vi "MainRTLocal.vi"() -> ()   [LabVIEW 2018]
doc: "The myRIO Project template acquires acceleration data from the onboard accelerometer and displays the changes of acceleration values in a waveform chart."
uses:
  <vilib>/myRIO/Instrument Drivers/Onboard IO/DIO/typedefs/DIO Reference.ctl
  <vilib>/myRIO/Common/Instrument Driver Framework/Utilities/typedefs/myRIO Generic Hardware Reference.ctl
  <vilib>/myRIO/Common/Instrument Driver Framework/Utilities/typedefs/Hardware Version Enum.ctl
  <vilib>/myRIO/Common/Instrument Driver Framework/Utilities/typedefs/myRIO v1.0 Reference.ctl
  <vilib>/myRIO/Common/Instrument Driver Framework/Utilities/typedefs/Generic FPGA Reference.ctl
  <vilib>/myRIO/Common/Instrument Driver Framework/myRIO v1.0/DIO/typedefs/DIO Channels List.ctl
  <vilib>/myRIO/Common/Instrument Driver Framework/myRIO v1.0/DIO/typedefs/DIO Channels Enum.ctl
  <vilib>/userdefined/High Color/nirio_resource_hc.ctl
  <vilib>/myRIO/Instrument Drivers/Onboard IO/PWM/typedefs/PWM Reference.ctl
  <vilib>/myRIO/Common/Instrument Driver Framework/myRIO v1.0/PWM/typedefs/PWM Channels Enum.ctl
  <vilib>/myRIO/Instrument Drivers/Onboard IO/PWM/typedefs/PWM Configuration.ctl
  <vilib>/myRIO/Common/Instrument Driver Framework/Utilities/vis/Is FPGA Ref Available.vi
  <vilib>/myRIO/Common/Instrument Driver Framework/myRIO v1.0/DIO/vis/myRIO v1.1 Open DIO.vi
  <vilib>/myRIO/Instrument Drivers/Onboard IO/DIO/vis/Write.vi
  <vilib>/myRIO/Common/Instrument Driver Framework/myRIO v1.0/PWM/vis/myRIO v1.1 Open PWM.vi
  <vilib>/myRIO/Instrument Drivers/Onboard IO/PWM/vis/Set Duty Cycle and Frequency.vi
  <vilib>/myRIO/Common/Instrument Driver Framework/Utilities/vis/Validate Channels.vi
  <vilib>/myRIO/Common/Instrument Driver Framework/myRIO v1.0/DIO/vis/myRIO v1.0 Reserve DIO.vi
  <vilib>/myRIO/Common/Instrument Driver Framework/myRIO v1.0/PWM/vis/myRIO v1.0 Reserve PWM.vi
  <vilib>/myRIO/Common/Instrument Driver Framework/myRIO v1.0/UART/vis/myRIO v1.0 Close UART.vi
  <vilib>/myRIO/Common/Instrument Driver Framework/myRIO v1.0/Resource Manager/vis/myRIO v1.0 Reserve Channel List.vi
  <vilib>/myRIO/Common/Instrument Driver Framework/myRIO v1.0/DIO/vis/myRIO v1.0 Build MUX Configuration DIO.vi
  <vilib>/myRIO/Common/Instrument Driver Framework/myRIO v1.0/PWM/vis/myRIO v1.0 Build MUX Configuration PWM.vi
  <vilib>/myRIO/Common/Instrument Driver Framework/myRIO v1.0/Resource Manager/vis/myRIO v1.0 Reserve Channel.vi
  <vilib>/myRIO/Common/Instrument Driver Framework/myRIO v1.0/Resource Manager/vis/myRIO v1.0 Unreserve Channel.vi
  <vilib>/myRIO/Common/Instrument Driver Framework/myRIO v1.0/Resource Manager/vis/myRIO v1.0 Create Configuration List.vi
  <vilib>/myRIO/Common/Instrument Driver Framework/myRIO v1.0/Resource Manager/vis/myRIO v1.0 Build Mutex Name.vi
  <vilib>/Utility/VariantDataType/GetNumericInfo.vi
  <vilib>/Utility/error.llb/Error Cluster From Error Code.vi
  <vilib>/myRIO/Common/Instrument Driver Framework/myRIO v1.0/myRIO v1.1 Open.vi
  <vilib>/myRIO/Common/Instrument Driver Framework/Utilities/vis/IO Manager.vi
  <vilib>/myRIO/Common/Instrument Driver Framework/Utilities/vis/Configuration Manager.vi
  <vilib>/myRIO/Common/Instrument Driver Framework/myRIO v1.0/Resource Manager/vis/myRIO v1.0 Configure IO.vi
  <vilib>/myRIO/Common/Instrument Driver Framework/myRIO v1.0/myRIO v1.0 Close.vi
  <vilib>/myRIO/Common/Instrument Driver Framework/myRIO v1.0/DIO/vis/myRIO v1.0 Write DIO.vi
  <vilib>/myRIO/Common/Instrument Driver Framework/myRIO v1.0/PWM/vis/myRIO v1.0 Write PWM.vi
  <vilib>/myRIO/Common/Instrument Driver Framework/Utilities/vis/FPGA Ref Manager.vi
  <vilib>/myRIO/Common/Instrument Driver Framework/myRIO v1.0/myRIO v1.0 Reset FPGA.vi
  <vilib>/myRIO/Common/Instrument Driver Framework/myRIO v1.0/IRQ/vis/myRIO v1.0 IRQ Info FGV.vi
  <vilib>/myRIO/Common/Instrument Driver Framework/myRIO v1.0/IRQ/vis/myRIO v1.0 Timer IRQ Info FGV.vi
  <vilib>/myRIO/Common/Instrument Driver Framework/myRIO v1.0/IRQ/vis/myRIO v1.0 ISR Agent.vi
  <vilib>/myRIO/Express VI/Onboard Devices/LED/LED Express VI.xnode
  <vilib>/myRIO/Instrument Drivers/Onboard IO/DIO/vis/myRIO DIO Open.xnode
  <vilib>/myRIO/Express VI/Onboard IO/PWM/PWM Express VI.xnode
  <vilib>/myRIO/Instrument Drivers/Onboard IO/PWM/vis/myRIO PWM Open.xnode
  <vilib>/myRIO/Instrument Drivers/Utilities/Utilities.lvlib
  <vilib>/myRIO/Instrument Drivers/Onboard IO/PWM/PWM.lvlib
  <vilib>/myRIO/Instrument Drivers/Onboard IO/DIO/DIO.lvlib
panel:
  out "LED0":bool
  in  "Frequency [Hz]":dbl(knob)=1000.0 scale=0.0..10000.0
  in  "Duty Cycle":dbl(slide)=0.5 scale=0.0..1.0
  out "error out":errorcluster
  in  "Stop":bool
  # "Overview: \nPWM Output Pin B/29 und GND B/28, blink LED0\nChange PWM frequency and duty cycle\nInstructions:\n1. Double click Express VI to change output channel\n2. Compare to MainRT for Network-Published Shared Variables"
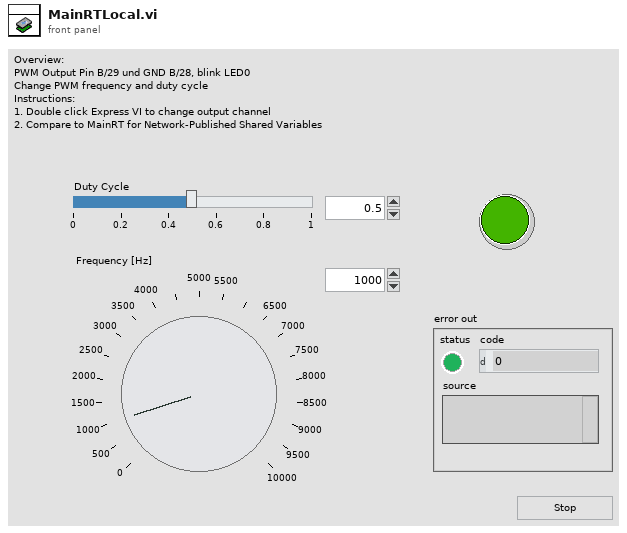
[diagram p1: front panel]
types:
  T1 = typedef "DIO.lvlib/DIO Reference.ctl" = cluster{"myRIO Reference":T2, "DIO Channels List":T6}
  T2 = typedef "myRIO Generic Hardware Reference.ctl" = cluster{"myRIO Model":T3, "myRIO Hardware Reference":T4}
  T3 = typedef "Hardware Version Enum.ctl" = enum16{"Unknown", "myRIO-1900", "myRIO-1950", "roboRIO", "NI ELVIS RIO CM", "ELVIS III"}
  T4 = typedef "myRIO v1.0 Reference.ctl" = cluster{"Generic FPGA Reference":T5, "Allow multiple opens":bool}
  T5 = typedef "Generic FPGA Reference.ctl" = refnum<k20>
  T6 = typedef "DIO Channels List.ctl" = T7[]
  T7 = typedef "DIO Channels Enum.ctl" = enum16{"Not Connected", "C/DIO0", "C/DIO1", "C/DIO2", "C/DIO3", "C/DIO4", "C/DIO5", "C/DIO6", "C/DIO7", "A/DIO0", "A/DIO1", "A/DIO2", "A/DIO3", "A/DIO4", "A/DIO5", "A/DIO6", "A/DIO7", "A/DIO8", "A/DIO9", "A/DIO10", "A/DIO11", "A/DIO12", "A/DIO13", "A/DIO14", "A/DIO15", "A/DIO16", "A/DIO17", "A/DIO18", "A/DIO19", "B/DIO0", "B/DIO1", "B/DIO2", "B/DIO3", "B/DIO4", "B/DIO5", "B/DIO6", "B/DIO7", "B/DIO8", "B/DIO9", "B/DIO10", "B/DIO11", "B/DIO12", "B/DIO13", "B/DIO14", "B/DIO15", "B/DIO16", "B/DIO17", "B/DIO18", "B/DIO19", "LED0", "LED1", "LED2", "LED3", "Button0", "DIO/DIO0", "DIO/DIO1", "DIO/DIO2", "DIO/DIO3", "DIO/DIO4", "DIO/DIO5", "DIO/DIO6", "DIO/DIO7", "DIO/DIO8", "DIO/DIO9", "SPI/CS0", "SPI/CS1", "SPI/CS2", "SPI/CS3", "LED RADIO (Green)", "LED RADIO (Red)", "LED COMM (Green)", "LED COMM (Red)", "LED MODE (Green)", "LED MODE (Red)"}
  T8 = typedef "nirio_resource_hc.ctl" = tag
  T9 = typedef "PWM.lvlib/PWM Reference.ctl" = cluster{"myRIO Reference":T2, "PWM Channels Enum":T10, "PWM Configuration":T11}
  T10 = typedef "PWM Channels Enum.ctl" = enum16{"Not Connected", "C/PWM0", "C/PWM1", "A/PWM0", "A/PWM1", "A/PWM2", "A/PWM3", "A/PWM4", "A/PWM5", "A/PWM6", "A/PWM7", "A/PWM8", "A/PWM9", "A/PWM10", "A/PWM11", "A/PWM12", "A/PWM13", "A/PWM14", "A/PWM15", "A/PWM16", "A/PWM17", "A/PWM18", "A/PWM19", "B/PWM0", "B/PWM1", "B/PWM2", "B/PWM3", "B/PWM4", "B/PWM5", "B/PWM6", "B/PWM7", "B/PWM8", "B/PWM9", "B/PWM10", "B/PWM11", "B/PWM12", "B/PWM13", "B/PWM14", "B/PWM15", "B/PWM16", "B/PWM17", "B/PWM18", "B/PWM19", "PWM/PWM0", "PWM/PWM1", "PWM/PWM2", "PWM/PWM3", "PWM/PWM4", "PWM/PWM5", "PWM/PWM6", "PWM/PWM7", "PWM/PWM8", "PWM/PWM9"}
  T11 = typedef "PWM.lvlib/PWM Configuration.ctl" = cluster{"Frequency":dbl, "Duty Cycle":dbl}
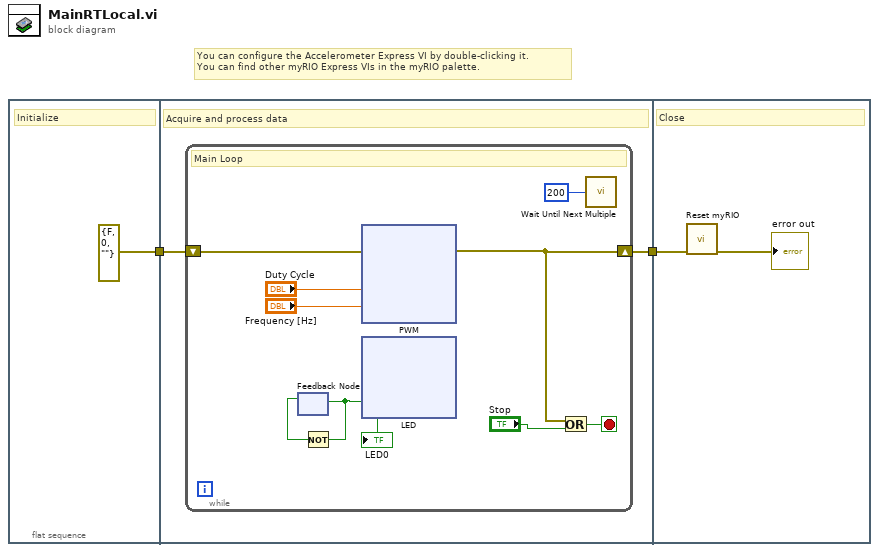
[diagram p0: block diagram]
diagram:
  # "You can configure the Accelerometer Express VI by double-clicking it.\nYou can find other myRIO Express VIs in the myRIO palette."
  n1 = flat-sequence {
    tunnel: [errorcluster {"status"=FALSE, "code"=0, "source"=""} ("error in (no error)")] -> w2
    tunnel: w2 -> [w5]
    tunnel: [w4] -> w1
    tunnel: w1 -> [w86]
    frame #0 {
      # "Initialize"
    }
    frame #1 {
      # "Acquire and process data"
      n2 = while {
        shift-right: [w12] -> w4
        shift-left: w5 -> [w13]
        stop <- w14 stop-if-true
        # "Main Loop"
        n3 = feedback #1() -> (w10:bool)  [unwired: 1 in]
        n4 = Not(x=w10) -> (.not. x?=w9:bool)
        "LED0" <- w9
        n5 = feedback-in #1(w9) -> ()
        n6 = xnode "PWM"("Duty Cycle"="Duty Cycle", "Frequency [Hz]"="Frequency [Hz]", "error in (no error)"=w13) -> ("error out"=w12:errorcluster)
        n7 = xnode "LED"("LED0"=w9) -> ()  [unwired: 1 in, 1 out]
        n8 = Or(x=w12, y="Stop") -> (x .or. y?=w14:bool)
        n9 = call "Wait Until Next Multiple"("Count(mSec)"=u32 200) -> ()  [unwired: 1 out]
      }
    }
    frame #2 {
      # "Close"
      n10 = call <vilib>:"Reset myRIO.vi"("error in (no error)"=w86) -> ("error out"=→"error out":errorcluster)  [unwired: 10 in]
    }
  }
